vi "Transmit - UDP (SAP).vi"() -> ()   [LabVIEW 2020]
uses:
  src/_controls/comm_config_vl_tx.ctl
  src/_controls/sap_config_tx.ctl
  src/helpers/EthFrameManagement/controls/mac_src_info_afdx.ctl
  src/_polimorphicInstances/session/Fdx Create Session (Tx-UDP Port-Oriented).vi
  src/bsp/AFDX_Transmit/Fdx Create Tx VL.vi
  src/_polimorphicInstances/udpPort/Fdx Create UDP Port (TX-SAP).vi
  src/_polimorphicInstances/control/Fdx Start (Tx).vi
  src/_polimorphicInstances/control/Fdx Stop (Tx).vi
  src/_polimorphicInstances/session/Fdx Close Session (Port).vi
  src/AIM664LV.lvlib
  src/helpers/EthFrameManagement/EthFrameManagement.lvlib
panel:
  in  "source info":T1
  in  "Period mS":u32=200
  in  "SapPort Config":T2={"partitionID"=0, "SubVlId"=0, "UdpSrcPort"=1, "UdpNumBufMessages"=0, "UdpMaxMessageSize"=1000}
  in  "VL Config":T3={"VlId"=30, "NumOfSubVl"=1, "rate mS (128)"=128.0, "domainID"=1, "sideID"=1, "locationID"=1, "interfaceID"=1, "NetSelect"=3, "Skew"=0, "MaxFrameLength"=1000, "FrameBufferSize"=0} {"NetSelect" items=["FDX_TX_FRAME_DLY_A"=0, "FDX_TX_FRAME_DLY_B"=1, "FDX_TX_FRAME_BOTH "=3, "FDX_TX_FRAME_ONLY_A"=4, "FDX_TX_FRAME_ONLY_B "=5]; "interfaceID" format="%.0b"}
  out "BytesWritten":u32
  out "current irig time":T4={"SignOut"=-1509901600, "DayOut"=16, "HourOut"=8, "MinOut"=7, "SecondOut"=53, "MilliSecOut"=368, "MicroSecOut"=508, "NanoSecOut"=600, "InfoOut"=0, "Mode"=3}
  out "CurrentIndex":u32
  out "MsgCount":u32
  out "IndexCycleCount":u32
  in  "VLid Dest":u32=30
  in  "UdpDst":u32=12345
  in  "Data":u8[](array[numeric])=[10, 10, 10, 10, 10, 10, 10, 10, 10, 10, 10, 10, 10, 10, 10, 10, 10, 10, 10, 10, 10, 10, 10, 10, 10, 10, 10, 10, 10, 10, 10, 10, 10, 10, 10, 10, 10, 10, 10, 10, 10, 10, 10, 10, 10, 10, 10, 10, 10, 10, 10, 10, 10, 10, 10, 10, 10, 10, 10, 10, 10, 10, 10, 10, 10, 10, 10, 10, 10, 10, 10, 10, 10, 10, 10, 10, 10, 10, 10, 10, 10, 10, 10, 10, 10, 10, 10, 10, 10, 10, 10, 10, 10, 10, 10, 10, 10, 10, 10, 15] format="%.0x"
  out "PortInitOut":T5={"PortConfig"=0, "PortUsed"=1, "GlobalMemFree"=0, "SharedMemFree"=0} {"PortConfig" items=["FDX_SINGLE", "FDX_REDUNDANT"]}
  in  "Port":u32
  in  "Board":u32=1
  out "error out":errorcluster
  in  "stop":bool
  out "current time":timestamp
  # "ARINC 664 Transmit UDP with Service Access Point (SAP)"
  # "Overview: Implements a Chronological Monitor for a specific Board and Port.\n\nRequirement: One AIM ARINC-664 board with installed AIM ARINC 664 BSP.\nRestrictions: None.\nInstruction:\n1. Select the Board ID (0 if you have only one board in your system).\n2. Run the VI.\n3. See the result in Current IRIG Time"
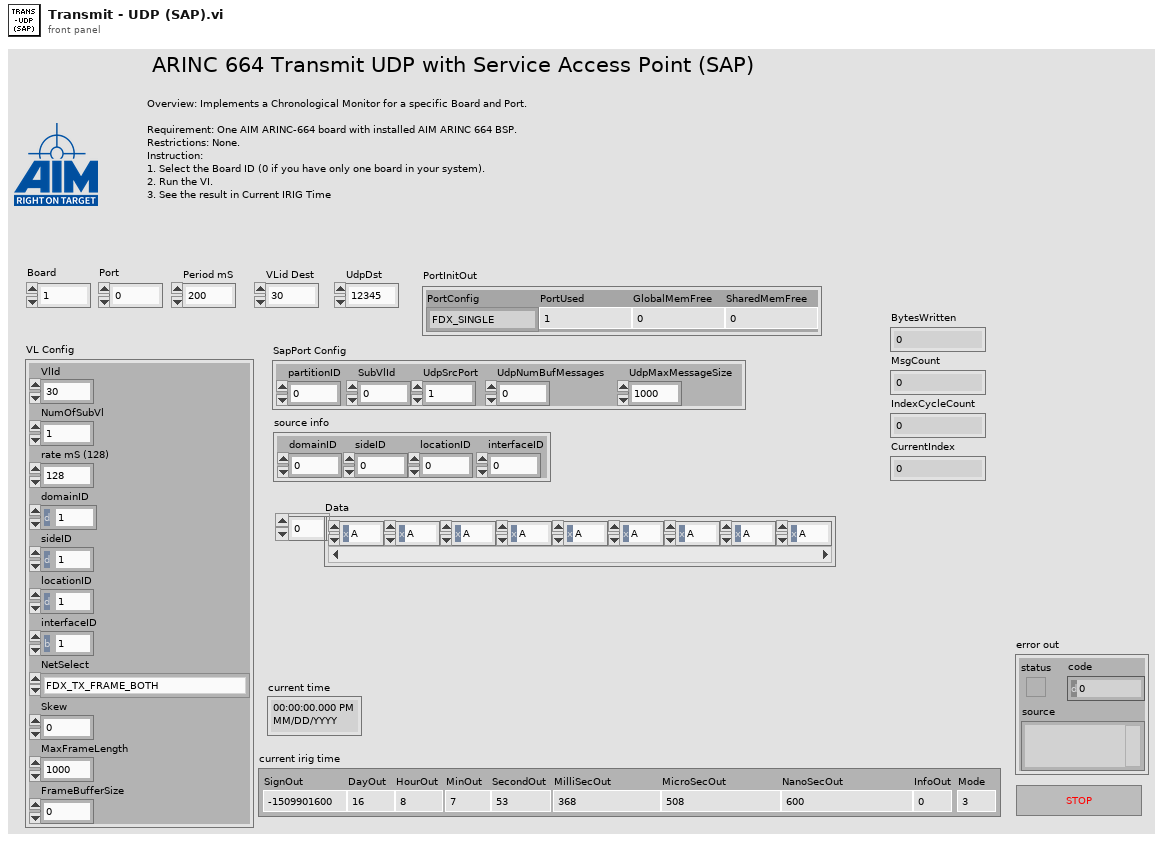
[diagram p1: front panel]
types:
  T1 = typedef "EthFrameManagement.lvlib/mac_src_info_afdx.ctl" = cluster{"domainID":u8, "sideID":u8, "locationID":u8, "interfaceID":u8}
  T2 = typedef "AIM664LV.lvlib/sap_config_tx.ctl" = cluster{"partitionID":u8, "SubVlId":u8, "UdpSrcPort":u16, "UdpNumBufMessages":u32, "UdpMaxMessageSize":u32}
  T3 = typedef "AIM664LV.lvlib/comm_config_vl_tx.ctl" = cluster{"VlId":u16, "NumOfSubVl":u16, "rate mS (128)":dbl, "domainID":u8, "sideID":u8, "locationID":u8, "interfaceID":u8, "NetSelect":u32, "Skew":u32, "MaxFrameLength":u32, "FrameBufferSize":u32}
  T4 = cluster{"SignOut":i32, "DayOut":u32, "HourOut":u32, "MinOut":u32, "SecondOut":u32, "MilliSecOut":u32, "MicroSecOut":u32, "NanoSecOut":u32, "InfoOut":u32, "Mode":u32}
  T5 = cluster{"PortConfig":u32, "PortUsed":u32, "GlobalMemFree":u32, "SharedMemFree":u32}
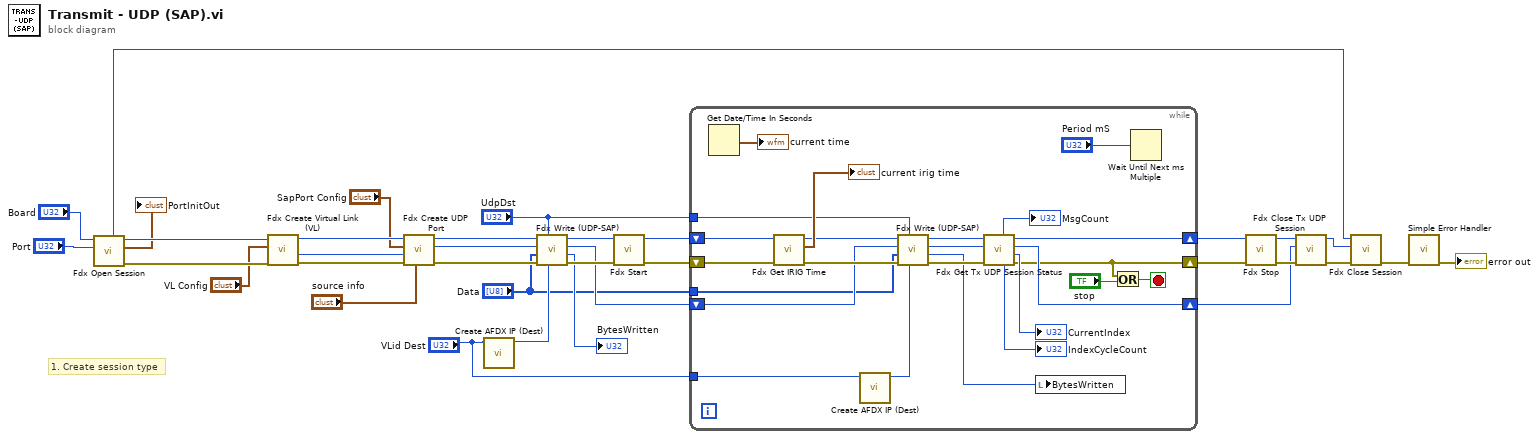
[diagram p0: block diagram]
diagram:
  # "1. Create session type"
  n1 = call-poly "Fdx Open Session.vi"("port"="Port", "board"="Board") -> ("error out"=w33:errorcluster, "PortInitOut"=→"PortInitOut":T5, "port handle out"=w34:u32, "InstrumentHandle_board out"=w9:u32)  [unwired: 5 in, 1 out]
  n2 = call-poly "Fdx Create Virtual Link (VL).vi"("error in (no error)"=w33, "VL Config"="VL Config", "InstrumentHandle in"=w34) -> ("error out"=w31:errorcluster, "VlId"=w21:u16, "InstrumentHandle out"=w32:u32)  [unwired: 6 in]
  n3 = call-poly "Fdx Create UDP Port.vi"("source info"="source info", "error in (no error)"=w31, "VlId"=w21, "SapPort Config"="SapPort Config", "port handle in"=w32) -> ("error out"=w24:errorcluster, "sapPort handle out"=w14:u32, "port handle out"=w17:u32)  [unwired: 3 in, 1 out]
  n4 = call "Create AFDX IP (Dest).vi"("VL"="VLid Dest") -> ("ip net"=w18:u32)  [unwired: 9 in, 1 out]
  n5 = call "Fdx Write (UDP-SAP).vi"("IpDst"=w18, "UdpDst"="UdpDst", "error in (no error)"=w24, "Data"="Data", "UdpHandle in"=w14, "InstrumentHandle_port in"=w17) -> ("error out"=w25:errorcluster, "BytesWritten"=→"BytesWritten":u32, "UdpHandle out"=w15:u32, "InstrumentHandle_port out"=w16:u32)  [unwired: 2 in]
  n6 = call-poly "Fdx Start.vi"("error in (no error)"=w25, "InstrumentHandle_port in"=w16) -> ("error out"=w7:errorcluster, "InstrumentHandle_port out"=w30:u32)  [unwired: 8 in]
  n7 = while {
    shift-right: [w45] -> w29
    shift-left: w30 -> [w55]
    shift-right: [w44] -> w12
    shift-left: w15 -> [w48]
    shift-right: [w39] -> w8
    shift-left: w7 -> [w35]
    tunnel: "Data" -> [w38]
    tunnel: "UdpDst" -> [w37]
    tunnel: "VLid Dest" -> [w36]
    stop <- w41 stop-if-true
    n8 = Get Date/Time In Seconds() -> (seconds since 1Jan1904=→"current time":timestamp)
    n9 = call "Fdx Get IRIG Time.vi"("error in (no error)"=w35, "InstrumentHandle_board in"=w55) -> ("error out"=w54:errorcluster, "Curent Irig Time"=→"current irig time":T4, "InstrumentHandle_board out"=w43:u32)  [unwired: 7 in]
    n10 = call "Create AFDX IP (Dest).vi"("VL"=w36) -> ("ip net"=w50:u32)  [unwired: 9 in, 1 out]
    n11 = call "Fdx Write (UDP-SAP).vi"("IpDst"=w50, "UdpDst"=w37, "error in (no error)"=w54, "Data"=w38, "UdpHandle in"=w48, "InstrumentHandle_port in"=w43) -> ("error out"=w52:errorcluster, "BytesWritten"=w49:u32, "UdpHandle out"=w47:u32, "InstrumentHandle_port out"=w51:u32)  [unwired: 2 in]
    n12 = call "Fdx Get Tx UDP Session Status.vi"("error in (no error)"=w52, "UdpHandle in"=w47, "InstrumentHandle_port in"=w51) -> ("error out"=w39:errorcluster, "CurrentIndex"=→"CurrentIndex":u32, "UdpHandle out"=w44:u32, "InstrumentHandle_port out"=w45:u32, "IndexCycleCount"=→"IndexCycleCount":u32, "MsgCount"=→"MsgCount":u32)  [unwired: 3 in]
    n13 = local write "BytesWritten"(w49) -> ()
    n14 = Or(x=w39, y="stop") -> (x .or. y?=w41:bool)
    n15 = Wait Until Next ms Multiple(millisecond multiple="Period mS") -> ()  [unwired: 1 out]
  }
  n16 = call-poly "Fdx Stop.vi"("error in (no error)"=w8, "InstrumentHandle_port in"=w29) -> ("error out"=w23:errorcluster, "InstrumentHandle_port out"=w11:u32)  [unwired: 8 in]
  n17 = call "Fdx Close Tx UDP Session.vi"("error in (no error)"=w23, "UdpHandle in"=w12, "InstrumentHandle_port in"=w11) -> ("error out"=w22:errorcluster, "InstrumentHandle_port out"=w10:u32)  [unwired: 7 in]
  n18 = call-poly "Fdx Close Session.vi"("error in (no error)"=w22, "InstrumentHandle_port in"=w10, "InstrumentHandle_board in"=w9) -> ("error out"=w2:errorcluster)  [unwired: 8 in]
  n19 = call <vilib>:"Simple Error Handler.vi"("error in (no error)"=w2) -> ("error out"=→"error out":errorcluster)  [unwired: 4 in, 4 out]
